vi "init.vi"(8 "error in (no error)":errorcluster, 11 "HP83623A_RF_Generator in":refnum<class "HP83623A_RF_Generator.lvclass">) -> (0 "error out":errorcluster, 3 "HP83623A_RF_Generator out":refnum<class "HP83623A_RF_Generator.lvclass">)   [LabVIEW 2013, in "HP83623A_RF_Generator.lvclass"]
uses:
  HP83623A_RF_Generator.lvclass
  HP83623A_array.ctl
  HP83623A.ctl
  HP83623A_RF_Generator.lvclass/HP83623A_RF_Generator.ctl
  Globals.vi
panel:
  out "HP83623A Generator Settings Array":T1
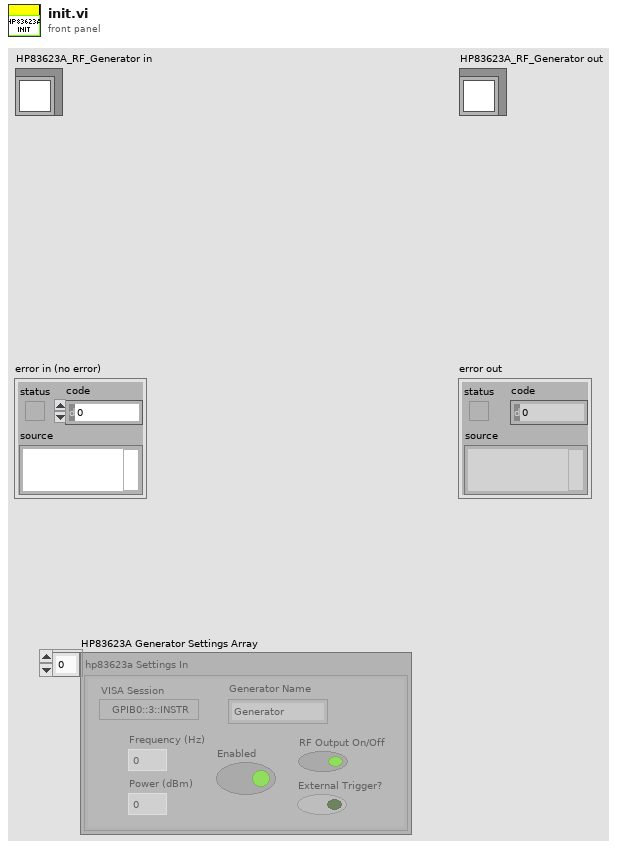
[diagram p1: front panel]
types:
  T1 = typedef "HP83623A_RF_Generator.lvclass/HP83623A_array.ctl" = T2[]
  T2 = typedef "HP83623A_RF_Generator.lvclass/HP83623A.ctl" = cluster{"Frequency (Hz)":dbl, "Power (dBm)":dbl, "Enabled":bool, "initialized":bool, "RF Output On/Off":bool, "External Trigger?":bool, "VISA Session":refnum<visa-resource-name>, "Generator Name":string}
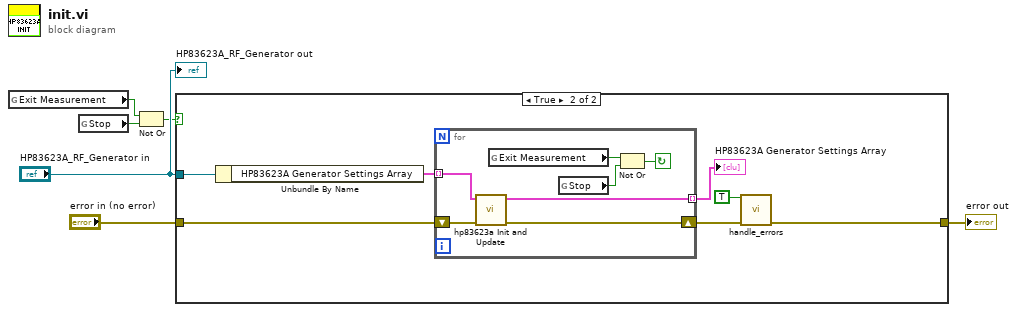
[diagram p0: block diagram]
diagram:
  n1 = global read "Globals.vi" "Exit Measurement"() -> (w3:bool)
  n2 = global read "Globals.vi" "Stop"() -> (w2:bool)
  n3 = Not Or(1:w2, 2:w3) -> (0:w1:bool)
  n4 = case shown="True" w1 {
    tunnel: "HP83623A_RF_Generator in" -> [_ w12]
    tunnel: "error in (no error)" -> [w7 w10]
    tunnel: [w7 w9] -> w4
    frame False {
    }
    frame True {
      n5 = Unbundle By Name(w12) -> ("HP83623A Generator Settings Array"=w11:T1)
      n6 = for {
        shift-right: [w20] -> w14
        shift-left: w10 -> [w21]
        tunnel: w11 -> [w19] mode=indexing
        tunnel: [w18] -> w13 mode=indexing
        stop <- w15 continue-if-true
        n7 = call "hp83623a Init and Update.vi"("error in (no error)"=w21, "hp83623a Settings (in)"=w19) -> ("error out"=w20:errorcluster, "hp83623a Settings"=w18:T2)  [unwired: 8 in]
        n8 = global read "Globals.vi" "Exit Measurement"() -> (w17:bool)
        n9 = global read "Globals.vi" "Stop"() -> (w16:bool)
        n10 = Not Or(1:w16, 2:w17) -> (0:w15:bool)
      }
      "HP83623A Generator Settings Array" <- w13
      n11 = call "handle_errors.vi"("Exit Operation"=TRUE, "error in (no error)"=w14) -> ("error out"=w9:errorcluster)  [unwired: 13 in]
    }
  }
  "error out" <- w4
  "HP83623A_RF_Generator out" <- "HP83623A_RF_Generator in"
